vi "user2.vi"() -> (0 "Numeric":dbl)   [LabVIEW 2021]
panel:
  in  "OK Button":bool
  in  "验证电压值[V]":dbl
  # "请填写验证电压值[V]"
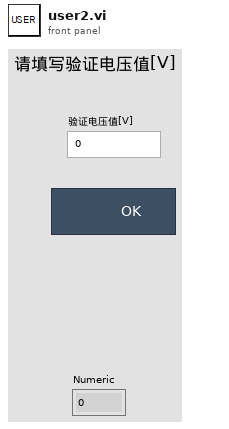
[diagram p1: front panel]
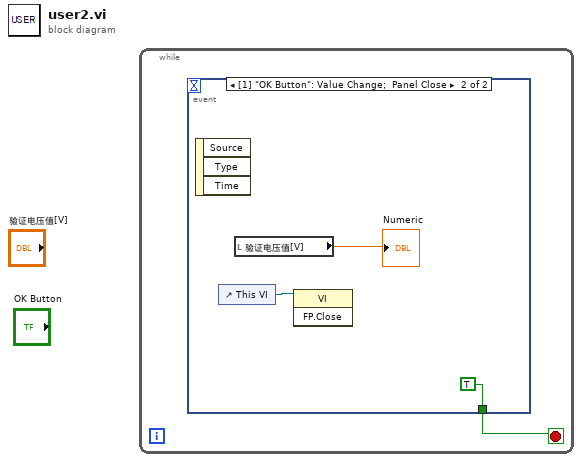
[diagram p0: block diagram]
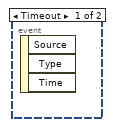
[diagram p2: hidden frame]
diagram:
  n1 = while {
    stop <- w1 stop-if-true
    n2 = event shown="[1] \"OK Button\": Value Change;  Panel Close" {
      selector: _ -> [_ _]
      dyn-events: _ -> [_ _]
      timeout: _ -> [_ _]
      tunnel: [_ TRUE] -> w1
      event Timeout {
        n3 = event-data() -> ()  [unwired: 1 in, 3 out]
      }
      event "OK Button": Value Change; Panel Close {
        n4 = event-data() -> ()  [unwired: 1 in, 3 out]
        n5 = control-ref of="This VI"() -> (w3:refnum<vi>)
        n6 = local read "验证电压值[V]"() -> (→"Numeric":dbl)
        n7 = invoke class="VI" method="FP.Close"(reference=w3) -> ()  [unwired: 2 in, 3 out]
      }
    }
  }
